vi "3.1.vi"(2 "x":dbl) -> (0 "sin":dbl, 1 "cos":dbl)   [LabVIEW 2017]
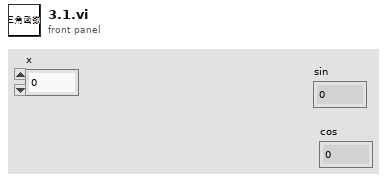
[diagram p1: front panel]
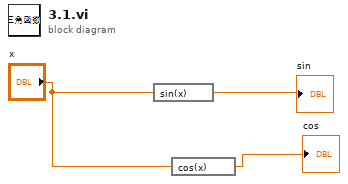
[diagram p0: block diagram]
diagram:
  n1 = expression code="sin(x)"("x") -> (→"sin":dbl)
  n2 = expression code="cos(x)"("x") -> (→"cos":dbl)
